vi "Configure Cells.vi"(8 "error in":errorcluster, 11 "tCRD in":refnum<class "Aircraft OPCCRD.lvclass">) -> (0 "error out":errorcluster, 3 "tCRD out":refnum<class "Aircraft OPCCRD.lvclass">)   [LabVIEW 2015, in "Aircraft OPCCRD.lvclass"]
uses:
  Aircraft OPCCRD.lvclass
  Reusable/CRDS/Cell/CRDS Cell.lvclass
  Reusable/CRDS/Data/Cell/CRDS Cell Data.lvclass
  Reusable/CRDS/Cell/Get Tau Method.ctl
  Data/tCRD Data.lvclass
  Aircraft OPCCRD.lvclass/Aircraft OPCCRD.ctl
  Reusable/Session APIs/File Access/Config Data/Config Data.lvclass/Config Data.ctl
  Reusable/CRDS/Cell/CRDS Cell.lvclass/CRDS Cell.ctl
  Reusable/Session APIs/File Access/Config Data/Accessors/Read Ref.vi
  Reusable/CRDS/Cell/Write Data.vi
  Reusable/CRDS/Cell/Write Nremove.vi
  Reusable/CRDS/Cell/Write NumTaus.vi
  <vilib>/Utility/config.llb/Read Key (Double).vi
  Reusable/General/Atmospheric/Atmospheric Constants.vi
  Reusable/CRDS/Cell/Write CalType.vi
  Reusable/CRDS/Cell/Write errorCalOn.vi
  Reusable/CRDS/Cell/Write dt.vi
  Reusable/CRDS/Cell/Write lambda.vi
  Reusable/CRDS/Cell/Write optTimeConst.vi
  Reusable/CRDS/Data/Main/Write CellData.vi
  Reusable/CRDS/Main/Write Data.vi
  Reusable/CRDS/Main/Write Cells.vi
  Reusable/General/Atmospheric/Atmospheric Library.lvlib
  Reusable/Session APIs/File Access/Config Data/Config Data.lvclass
  <vilib>/Utility/config.llb/NI_LVConfig.lvlib
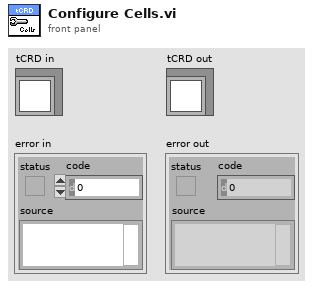
[diagram p1: front panel]
types:
  T1 = typedef "Get Tau Method.ctl" = enum8{"DFT-1", "DFT-5", "LRS"}
  T2 = typedef "Config Data.lvclass/Config Session.ctl" = refnum<data-value>
  T3 = typedef "NI_LVConfig.lvlib/Config Data RefNum.ctl" = refnum<k1>
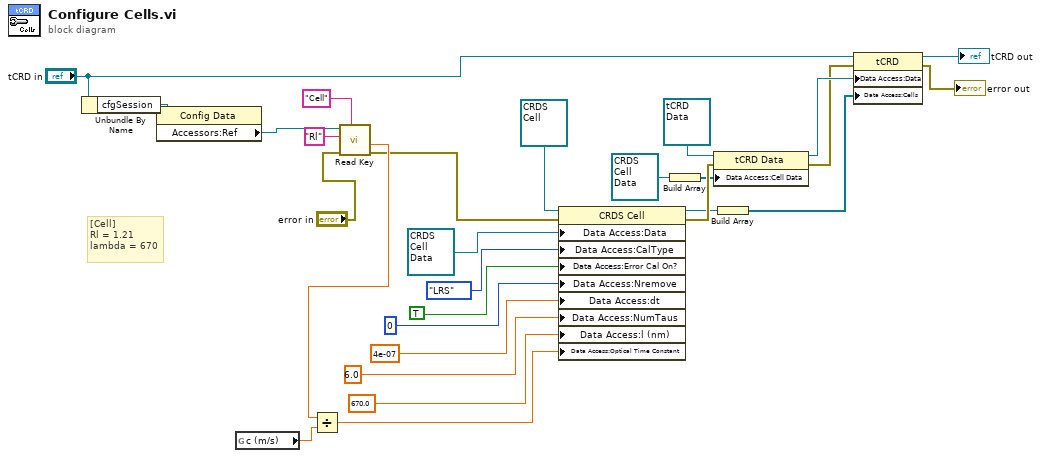
[diagram p0: block diagram]
diagram:
  # "[Cell]\nRl = 1.21\nlambda = 670"
  n1 = Unbundle By Name("tCRD in") -> ("cfgSession"=w7:T2)
  n2 = property class="Config Data"(reference=w7) -> ("Accessors:Ref"=w6:T3)  [unwired: 1 in, 2 out]
  n3 = global read "Atmospheric Constants.vi" "c (m/s)"() -> (w15:dbl)
  n4 = call-poly <vilib>:"Read Key.vi"("section"="Cell", "error in (no error)"="error in", "key"="Rl", "refnum"=w6) -> ("error out"=w1:errorcluster, "value"=w3:dbl)  [unwired: 4 in, 2 out]
  n5 = Divide(x=w3, y=w15) -> (x/y=w14:dbl)
  n6 = property class="CRDS Cell"(reference=refnum<class "CRDS Cell.lvclass"> refnum ("CRDS Cell"), error in=w1, "Data Access:Data"=refnum<class "CRDS Cell Data.lvclass"> refnum ("Data"), "Data Access:CalType"=Get_Tau_Method."LRS" ("CalType"), "Data Access:Error Cal On?"=TRUE ("Error Cal On?"), "Data Access:Nremove"=0 ("Nremove"), "Data Access:dt"=4e-07 ("dt"), "Data Access:NumTaus"=sgl 6.0 ("NumTaus"), "Data Access:l (nm)"=sgl 670.0 ("l (nm)"), "Data Access:Optical Time Constant"=w14) -> (reference out=w23:refnum<class "CRDS Cell.lvclass">, error out=w25:errorcluster)
  n7 = Build Array(refnum<class "CRDS Cell Data.lvclass"> refnum ("CRDS Cell Data.lvclass")) -> (w18:refnum<class "CRDS Cell Data.lvclass">[])
  n8 = property class="tCRD Data"(reference=refnum<class "tCRD Data.lvclass"> refnum ("tCRD Data"), error in=w25, "Data Access:Cell Data"=w18) -> (reference out=w12:refnum<class "tCRD Data.lvclass">, error out=w10:errorcluster)
  n9 = Build Array(w23) -> (w11:refnum<class "CRDS Cell.lvclass">[])
  n10 = property class="tCRD"(reference="tCRD in", error in=w10, "Data Access:Data"=w12, "Data Access:Cells"=w11) -> (reference out=→"tCRD out":refnum<class "Aircraft OPCCRD.lvclass">, error out=→"error out":errorcluster)
